vi "LV3Climb.vi"(7 "Deactivate?":bool, 8 "error in (no error)":errorcluster, 9 "Activate?":bool, 10 "Reclimb?":bool, 11 "Elevator Concrete in":refnum<class "Elevator Arm.lvclass">) -> (0 "error out":errorcluster, 1 "activate wrist lock":bool, 3 "Elevator Concrete out":refnum<class "Elevator Arm.lvclass">)   [LabVIEW 2018, in "Elevator.lvlib" / "Elevator Arm.lvclass"]
uses:
  Elevator Arm.lvclass
  C:/Users/Howdy Bots/Documents/2019DeepSpace/Classes/Elevator/Elevator.lvclass
  Controls/Elevator States Climb.ctl
  Elevator.lvclass/Elevator.ctl
  <vilib>/Rock Robotics/WPI/ThirdParty/Phoenix-LabVIEW/Motor Controller/Controls/CTRE_Phoenix_MotorControl_ControlMode.ctl
  Elevator Arm.lvclass/Elevator Arm.ctl
  Public Methods/Read Arm Position Values.vi
  <vilib>/Rock Robotics/WPI/ThirdParty/Phoenix-LabVIEW/Motor Controller/Get/CTRE_Phoenix_MotorController_GetQuadratureData.vi
  <vilib>/Rock Robotics/Network Tables/NT Write String.vi
  Elevator.lvclass
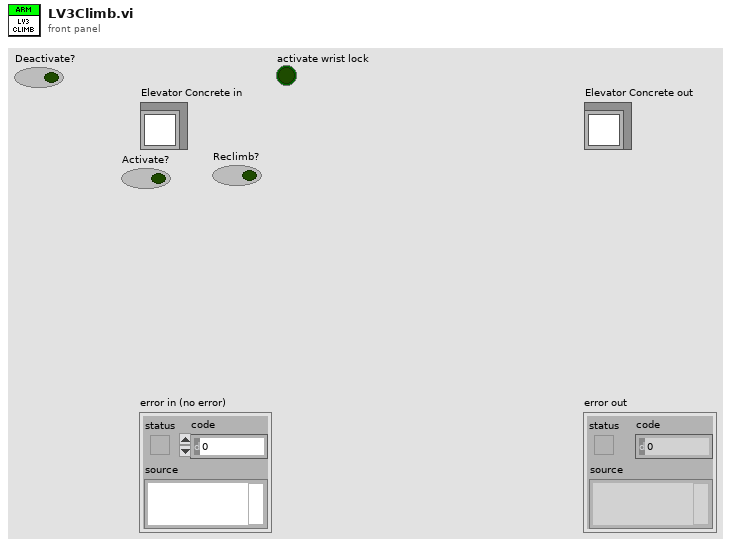
[diagram p1: front panel]
types:
  T1 = typedef "Elevator.lvlib/Elevator.lvclass/Elevator States Climb.ctl" = enum16{"Pre-Lift", "Deploy", "Activate Suction", "Climb", "Climbed", "Unclimb", ""}
  T2 = typedef "Elevator.lvlib/Elevator.lvclass/Elevator Constants.ctl" = cluster{"Arm Motion Magic Max Velocity":u32, "Arm Motion Magic Max Acceleration":u32, "Wrist Motion Magic Max Velocity":u32, "Wrist Motion Magic Max Acceleration":u32, "Elevator Linear Motion Magic Max Velocity":u32, "Elevator Linear Motion Magic Max Acceleration":u32, "Arm Gear Ratio":dbl, "Wrist Gear Ratio":dbl, "Elevator Linear Gear Ratio":dbl, "Arm Encoder ABS Value":i32, "Wrist Encoder ABS Value":i32}
  T3 = typedef "Elevator.lvlib/Elevator.lvclass/Arm Position Values.ctl" = cluster{"C0 Arm":dbl, "C1 Arm":dbl, "C2 Arm":dbl, "H1 Arm":dbl, "H2 Arm":dbl, "C0 Wrist":dbl, "C1 Wrist ":dbl, "C2 Wrist":dbl, "H1 Wrist":dbl, "H2 Wrist":dbl, "Deploy Arm":dbl, "Deploy Wrist":dbl, "Climb Arm":dbl, "Climb Wrist":dbl, "Stowed Arm":dbl, "Stowed Wrist":dbl, "CS":dbl, "C0":dbl, "C1":dbl, "C2":dbl, "C3":dbl, "H0":dbl, "H1":dbl, "H2":dbl}
  T4 = typedef "CTRE_Phoenix_MotorControl_ControlMode.ctl" = u16
  T5 = typedef "WPI_MotorControlDeviceRef.ctl" = cluster{"DeviceStatus":errorcluster, "Type":T6, "PWM":cluster{"PWM Channel":T7, "DeadBand":T8}, "CAN":cluster{"Device Number":u8, "SetOutput VI Ref":variant, "GetOutput VI Ref":variant, "Enable VI Ref":variant, "Disable VI Ref":variant, "Data":variant}, "Invert":bool, "DIO PWM":cluster{"PWM \"Enable\" Channel":T7, "DIOChannel":T9, "PWM Rate":dbl}}
  T6 = typedef "WPI_MotorControlType.ctl" = enum16{"PWM", "CAN", "DIO PWM"}
  T7 = typedef "FPGA_DIOPWMChannel.ctl" = enum8{"PWM 0", "PWM 1", "PWM 2", "PWM 3", "PWM 4", "PWM 5", "PWM 6", "PWM 7", "PWM 8", "PWM 9", "PWM MXP 0", "PWM MXP 1", "PWM MXP 2", "PWM MXP 3", "PWM MXP 4", "PWM MXP 5", "PWM MXP 6", "PWM MXP 7", "PWM MXP 8", "PWM MXP 9", "Invalid"}
  T8 = typedef "WPI_PWMDeadband.ctl" = cluster{"Name":string, "maxPositivePwm":i32, "minPositivePwm":i32, "centerPwm":i32, "maxNegativePwm":i32, "minNegativePwm":i32, "angularRange":u16}
  T9 = typedef "FPGA_DIOChannel.ctl" = enum8{"DIO 0", "DIO 1", "DIO 2", "DIO 3", "DIO 4", "DIO 5", "DIO 6", "DIO 7", "DIO 8", "DIO 9", "DIO MXP 0", "DIO MXP 1", "DIO MXP 2", "DIO MXP 3", "DIO MXP 4", "DIO MXP 5", "DIO MXP 6", "DIO MXP 7", "DIO MXP 8", "DIO MXP 9", "DIO MXP 10", "DIO MXP 11", "DIO MXP 12", "DIO MXP 13", "DIO MXP 14", "DIO MXP 15", "SPI Port CS1", "SPI Port CS2", "SPI Port CS3", "SPI Port MISO", "SPI Port MOSI", "Invalid"}
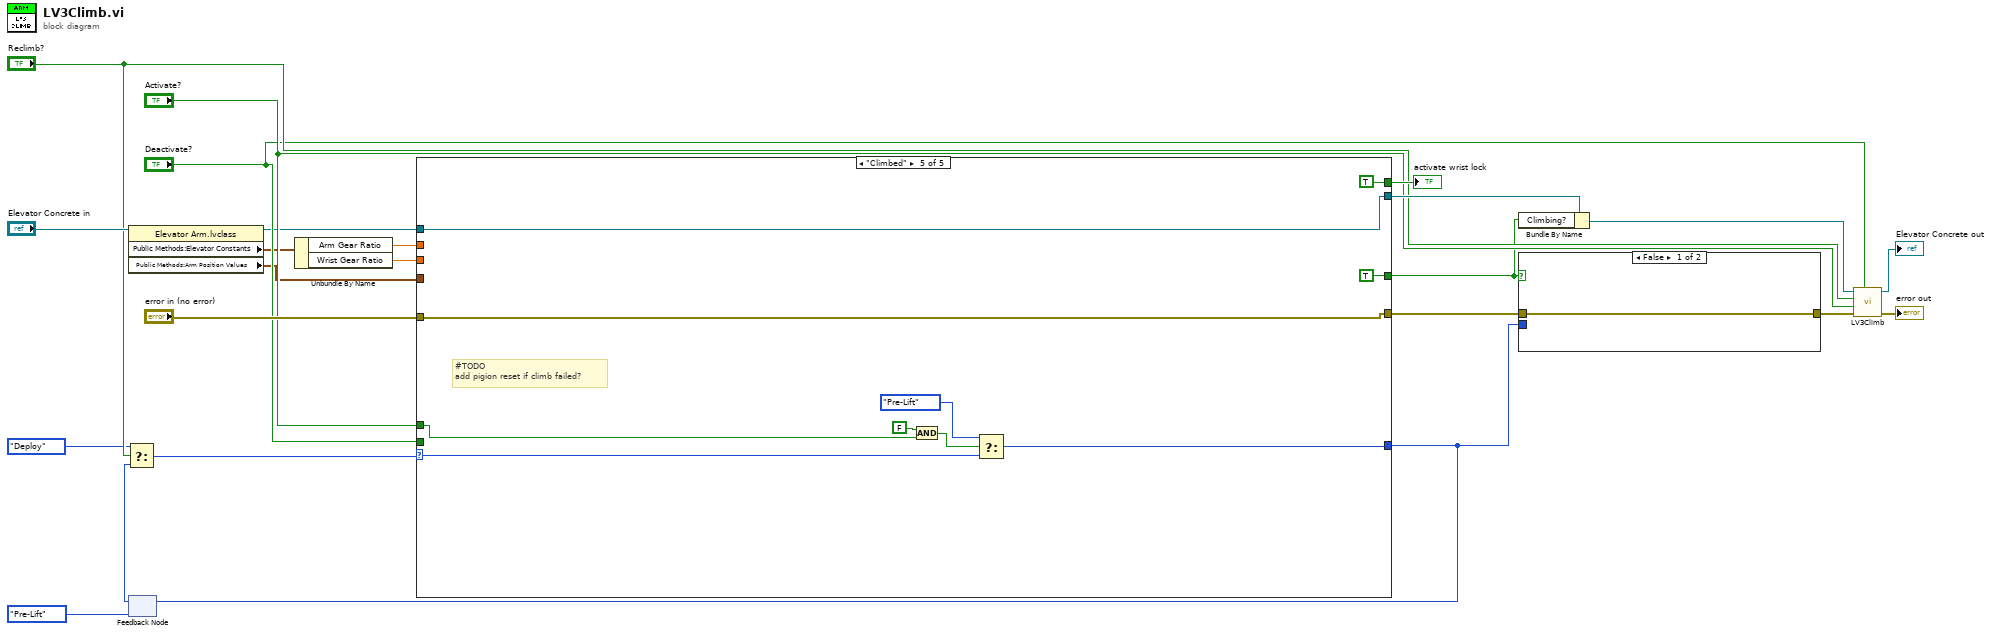
[diagram p0: block diagram]
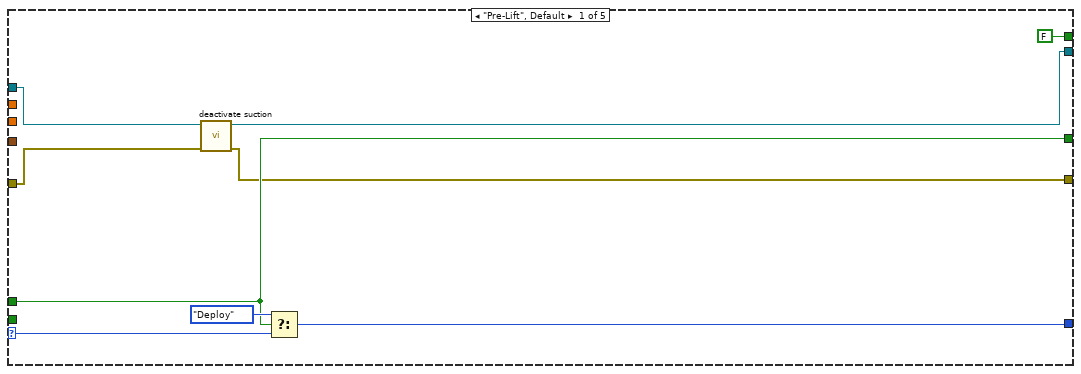
[diagram p2: hidden frame]
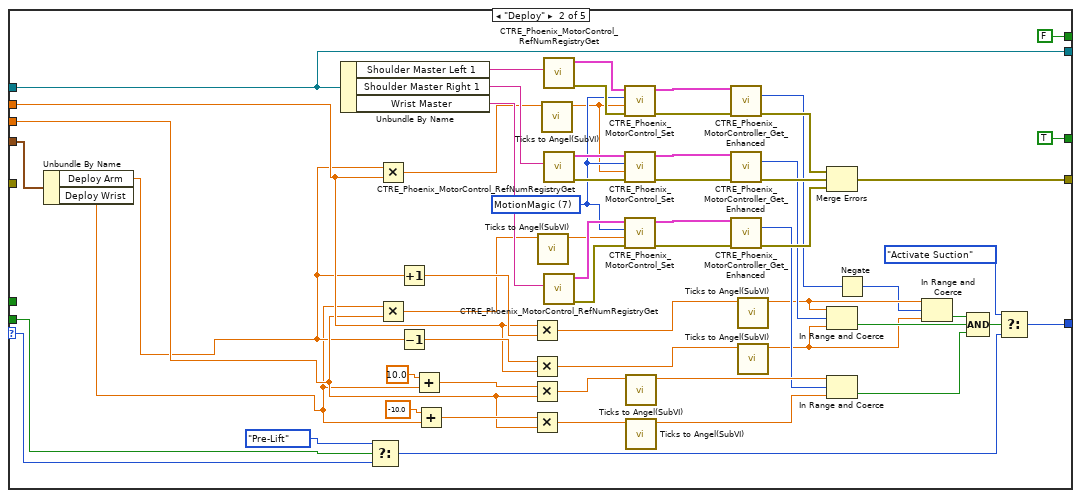
[diagram p3: hidden frame]
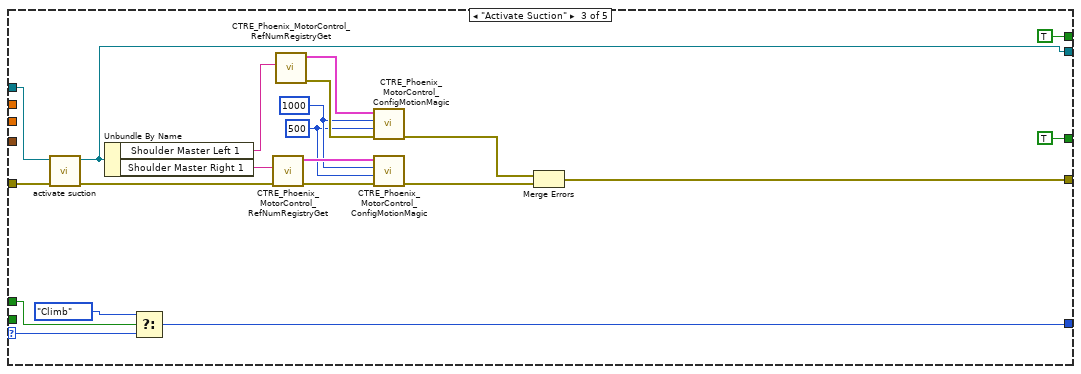
[diagram p4: hidden frame]
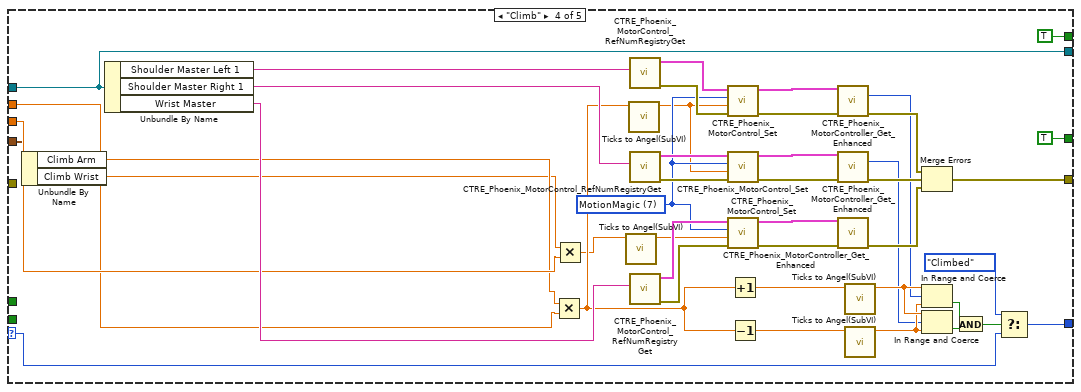
[diagram p5: hidden frame]
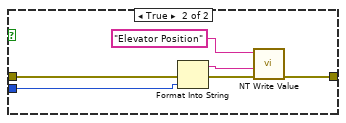
[diagram p6: hidden frame]
diagram:
  n1 = property class="Elevator Arm.lvclass"(reference="Elevator Concrete in") -> (reference out=w5:refnum<class "Elevator Arm.lvclass">, "Public Methods:Elevator Constants"=w3:T2, "Public Methods:Arm Position Values"=w4:T3)  [unwired: 1 in, 1 out]
  n2 = feedback #1(Elevator_States_Climb."Pre-Lift") -> (w13:T1)
  n3 = Select(t=Elevator_States_Climb."Deploy", s="Reclimb?", f=w13) -> (s? t:f=w7:T1)
  n4 = Unbundle By Name(w3) -> ("Arm Gear Ratio"=w2:dbl, "Wrist Gear Ratio"=w1:dbl)
  n5 = case shown="\"Climbed\"" w7 {
    selector: w7 -> [w31 w38 w110 w157 w160]
    tunnel: "Activate?" -> [w29 _ w107 _ w164]
    tunnel: w5 -> [w27 w92 w113 w152 w167]
    tunnel: [w26 w92 w106 w152 w167] -> w22
    tunnel: "error in (no error)" -> [w25 _ w112 _ w166]
    tunnel: [w24 w91 w98 w155 w166] -> w11
    tunnel: [w30 w90 w111 w156 w161] -> w9
    tunnel: [w29 TRUE TRUE TRUE TRUE] -> w8
    tunnel: [FALSE FALSE TRUE TRUE TRUE] -> w19
    tunnel: "Deactivate?" -> [_ w40 _ _ _]
    tunnel: w4 -> [_ w35 _ w116 _]
    tunnel: w2 -> [_ w37 _ w117 _]
    tunnel: w1 -> [_ w36 _ w118 _]
    frame "Pre-Lift", Default {
      n6 = call "deactivate suction.vi"("error in (no error)"=w25, "Elevator Concrete in"=w27) -> ("error out"=w24:errorcluster, "Elevator Concrete out"=w26:refnum<class "Elevator Arm.lvclass">)  [unwired: 8 in]
      n7 = Select(t=Elevator_States_Climb."Deploy", s=w29, f=w31) -> (s? t:f=w30:T1)
    }
    frame "Deploy" {
      w68 = T4 7 items=["PercentOutput"=0, "Position"=1, "Velocity"=2, "Current"=3, "Follower"=5, "MotionProfile"=6, "MotionMagic"=7, "MotionProfileArc"=10, "Disabled"=15] ("Control Mode")
      n8 = Unbundle By Name(w35) -> ("Deploy Arm"=w34:dbl, "Deploy Wrist"=w33:dbl)
      n9 = Unbundle By Name(w92) -> ("Shoulder Master Left 1"=w67:string, "Shoulder Master Right 1"=w82:string, "Wrist Master"=w83:string)
      n10 = Select(t=Elevator_States_Climb."Pre-Lift", s=w40, f=w38) -> (s? t:f=w39:T1)
      n11 = Multiply(x=w34, y=w37) -> (x*y=w45:dbl)
      n12 = Multiply(x=w33, y=w36) -> (x*y=w50:dbl)
      n13 = Increment(x=w34) -> (x+1=w60:dbl)
      n14 = Decrement(x=w34) -> (x-1=w59:dbl)
      n15 = Add(x=10.0, y=w33) -> (x+y=w57:dbl)
      n16 = Add(x=-10.0, y=w33) -> (x+y=w56:dbl)
      n17 = Multiply(x=w37, y=w60) -> (x*y=w43:dbl)
      n18 = Multiply(x=w59, y=w37) -> (x*y=w44:dbl)
      n19 = Multiply(x=w57, y=w36) -> (x*y=w47:dbl)
      n20 = Multiply(x=w56, y=w36) -> (x*y=w46:dbl)
      n21 = call "Ticks to Angel(SubVI).vi"("Numeric in"=w50) -> ("Numeric out"=w73:dbl)  [unwired: 10 in]
      n22 = call "Ticks to Angel(SubVI).vi"("Numeric in"=w45) -> ("Numeric out"=w65:dbl)  [unwired: 10 in]
      n23 = call <vilib>:"CTRE_Phoenix_MotorControl_RefNumRegistryGet.vi"("refnum name"=w67) -> ("error out"=w70:errorcluster, "PhoenixMotorControlDevRef"=w72:T5)  [unwired: 9 in]
      n24 = call <vilib>:"CTRE_Phoenix_MotorControl_RefNumRegistryGet.vi"("refnum name"=w82) -> ("error out"=w87:errorcluster, "PhoenixMotorControlDevRef"=w86:T5)  [unwired: 9 in]
      n25 = call <vilib>:"CTRE_Phoenix_MotorControl_RefNumRegistryGet.vi"("refnum name"=w83) -> ("error out"=w84:errorcluster, "PhoenixMotorControlDevRef"=w85:T5)  [unwired: 9 in]
      n26 = call <vilib>:"CTRE_Phoenix_MotorControl_Set.vi"("error in (no error)"=w70, "Output"=w65, "Control Mode"=w68, "PhoenixMotorControlDevRef"=w72) -> ("error out"=w69:errorcluster, "PhoenixMotorControlDevRef"=w71:T5)  [unwired: 6 in]
      n27 = call <vilib>:"CTRE_Phoenix_MotorControl_Set.vi"("error in (no error)"=w87, "Output"=w65, "Control Mode"=w68, "PhoenixMotorControlDevRef"=w86) -> ("error out"=w77:errorcluster, "PhoenixMotorControlDevRef"=w78:T5)  [unwired: 6 in]
      n28 = call <vilib>:"CTRE_Phoenix_MotorControl_Set.vi"("error in (no error)"=w84, "Output"=w73, "Control Mode"=w68, "PhoenixMotorControlDevRef"=w85) -> ("error out"=w79:errorcluster, "PhoenixMotorControlDevRef"=w80:T5)  [unwired: 6 in]
      n29 = call "Ticks to Angel(SubVI).vi"("Numeric in"=w47) -> ("Numeric out"=w54:dbl)  [unwired: 10 in]
      n30 = call "Ticks to Angel(SubVI).vi"("Numeric in"=w46) -> ("Numeric out"=w55:dbl)  [unwired: 10 in]
      n31 = call-poly <vilib>:"CTRE_Phoenix_MotorController_Get_Enhanced.vi"("PhoenixMotorControlDevRef"=w71, "error in"=w69) -> ("Quadrature Position"=w61:i32, "error out"=w66:errorcluster)  [unwired: 10 in, 2 out]
      n32 = call-poly <vilib>:"CTRE_Phoenix_MotorController_Get_Enhanced.vi"("PhoenixMotorControlDevRef"=w78, "error in"=w77) -> ("Quadrature Position"=w58:i32, "error out"=w75:errorcluster)  [unwired: 10 in, 2 out]
      n33 = call-poly <vilib>:"CTRE_Phoenix_MotorController_Get_Enhanced.vi"("PhoenixMotorControlDevRef"=w80, "error in"=w79) -> ("Quadrature Position"=w53:i32, "error out"=w74:errorcluster)  [unwired: 10 in, 2 out]
      n34 = call "Ticks to Angel(SubVI).vi"("Numeric in"=w43) -> ("Numeric out"=w52:dbl)  [unwired: 10 in]
      n35 = call "Ticks to Angel(SubVI).vi"("Numeric in"=w44) -> ("Numeric out"=w51:dbl)  [unwired: 10 in]
      n36 = Merge Errors(w66, w75, w74) -> (w91:errorcluster)
      n37 = In Range and Coerce(upper limit=w52, x=w58, lower limit=w51) -> (In Range?=w63:bool)  [unwired: 1 out]
      n38 = In Range and Coerce(upper limit=w54, x=w53, lower limit=w55) -> (In Range?=w64:bool)  [unwired: 1 out]
      n39 = Negate(x=w61) -> (-x=w42:i32)
      n40 = In Range and Coerce(upper limit=w52, x=w42, lower limit=w51) -> (In Range?=w62:bool)  [unwired: 1 out]
      n41 = Compound Arithmetic op=AND(w62, w63, w64) -> (w76:bool)
      n42 = Select(t=Elevator_States_Climb."Activate Suction", s=w76, f=w39) -> (s? t:f=w90:T1)
    }
    frame "Activate Suction" {
      w95 = 1000 ("Cruise Velocity")
      w94 = 500 ("Acceleration")
      n43 = call "activate suction.vi"("error in (no error)"=w112, "Elevator Concrete in"=w113) -> ("error out"=w99:errorcluster, "Elevator Concrete out"=w106:refnum<class "Elevator Arm.lvclass">)  [unwired: 8 in]
      n44 = Unbundle By Name(w106) -> ("Shoulder Master Left 1"=w104:string, "Shoulder Master Right 1"=w105:string)
      n45 = Select(t=Elevator_States_Climb."Climb", s=w107, f=w110) -> (s? t:f=w111:T1)
      n46 = call <vilib>:"CTRE_Phoenix_MotorControl_RefNumRegistryGet.vi"("error in (no error)"=w99, "refnum name"=w105) -> ("error out"=w103:errorcluster, "PhoenixMotorControlDevRef"=w102:T5)  [unwired: 8 in]
      n47 = call <vilib>:"CTRE_Phoenix_MotorControl_RefNumRegistryGet.vi"("refnum name"=w104) -> ("error out"=w101:errorcluster, "PhoenixMotorControlDevRef"=w100:T5)  [unwired: 9 in]
      n48 = call <vilib>:"CTRE_Phoenix_MotorControl_ConfigMotionMagic.vi"("error in (no error)"=w101, "Acceleration"=w94, "Cruise Velocity"=w95, "PhoenixMotorControlDevRef"=w100) -> ("error out"=w97:errorcluster)  [unwired: 6 in, 1 out]
      n49 = call <vilib>:"CTRE_Phoenix_MotorControl_ConfigMotionMagic.vi"("error in (no error)"=w103, "Acceleration"=w94, "Cruise Velocity"=w95, "PhoenixMotorControlDevRef"=w102) -> ("error out"=w96:errorcluster)  [unwired: 6 in, 1 out]
      n50 = Merge Errors(w97, w96) -> (w98:errorcluster)
    }
    frame "Climb" {
      w134 = T4 7 items=["PercentOutput"=0, "Position"=1, "Velocity"=2, "Current"=3, "Follower"=5, "MotionProfile"=6, "MotionMagic"=7, "MotionProfileArc"=10, "Disabled"=15] ("Control Mode")
      n51 = Unbundle By Name(w116) -> ("Climb Arm"=w115:dbl, "Climb Wrist"=w114:dbl)
      n52 = Unbundle By Name(w152) -> ("Shoulder Master Left 1"=w133:string, "Shoulder Master Right 1"=w146:string, "Wrist Master"=w147:string)
      n53 = Multiply(x=w115, y=w117) -> (x*y=w120:dbl)
      n54 = Multiply(x=w114, y=w118) -> (x*y=w119:dbl)
      n55 = call "Ticks to Angel(SubVI).vi"("Numeric in"=w119) -> ("Numeric out"=w121:dbl)  [unwired: 10 in]
      n56 = call "Ticks to Angel(SubVI).vi"("Numeric in"=w120) -> ("Numeric out"=w122:dbl)  [unwired: 10 in]
      n57 = call <vilib>:"CTRE_Phoenix_MotorControl_RefNumRegistryGet.vi"("refnum name"=w133) -> ("error out"=w136:errorcluster, "PhoenixMotorControlDevRef"=w138:T5)  [unwired: 9 in]
      n58 = call <vilib>:"CTRE_Phoenix_MotorControl_RefNumRegistryGet.vi"("refnum name"=w146) -> ("error out"=w151:errorcluster, "PhoenixMotorControlDevRef"=w150:T5)  [unwired: 9 in]
      n59 = call <vilib>:"CTRE_Phoenix_MotorControl_RefNumRegistryGet.vi"("refnum name"=w147) -> ("error out"=w148:errorcluster, "PhoenixMotorControlDevRef"=w149:T5)  [unwired: 9 in]
      n60 = call <vilib>:"CTRE_Phoenix_MotorControl_Set.vi"("error in (no error)"=w136, "Output"=w122, "Control Mode"=w134, "PhoenixMotorControlDevRef"=w138) -> ("error out"=w135:errorcluster, "PhoenixMotorControlDevRef"=w137:T5)  [unwired: 6 in]
      n61 = call <vilib>:"CTRE_Phoenix_MotorControl_Set.vi"("error in (no error)"=w151, "Output"=w122, "Control Mode"=w134, "PhoenixMotorControlDevRef"=w150) -> ("error out"=w142:errorcluster, "PhoenixMotorControlDevRef"=w143:T5)  [unwired: 6 in]
      n62 = call <vilib>:"CTRE_Phoenix_MotorControl_Set.vi"("error in (no error)"=w148, "Output"=w121, "Control Mode"=w134, "PhoenixMotorControlDevRef"=w149) -> ("error out"=w144:errorcluster, "PhoenixMotorControlDevRef"=w145:T5)  [unwired: 6 in]
      n63 = Increment(x=w120) -> (x+1=w130:dbl)
      n64 = Decrement(x=w120) -> (x-1=w129:dbl)
      n65 = call-poly <vilib>:"CTRE_Phoenix_MotorController_Get_Enhanced.vi"("PhoenixMotorControlDevRef"=w137, "error in"=w135) -> ("Quadrature Position"=w125:i32, "error out"=w132:errorcluster)  [unwired: 10 in, 2 out]
      n66 = call-poly <vilib>:"CTRE_Phoenix_MotorController_Get_Enhanced.vi"("PhoenixMotorControlDevRef"=w143, "error in"=w142) -> ("Quadrature Position"=w126:i32, "error out"=w140:errorcluster)  [unwired: 10 in, 2 out]
      n67 = call-poly <vilib>:"CTRE_Phoenix_MotorController_Get_Enhanced.vi"("PhoenixMotorControlDevRef"=w145, "error in"=w144) -> ("error out"=w139:errorcluster)  [unwired: 10 in, 3 out]
      n68 = call "Ticks to Angel(SubVI).vi"("Numeric in"=w130) -> ("Numeric out"=w128:dbl)  [unwired: 10 in]
      n69 = call "Ticks to Angel(SubVI).vi"("Numeric in"=w129) -> ("Numeric out"=w127:dbl)  [unwired: 10 in]
      n70 = Merge Errors(w132, w140, w139) -> (w155:errorcluster)
      n71 = In Range and Coerce(upper limit=w128, x=w125, lower limit=w127) -> (In Range?=w123:bool)  [unwired: 1 out]
      n72 = In Range and Coerce(upper limit=w128, x=w126, lower limit=w127) -> (In Range?=w124:bool)  [unwired: 1 out]
      n73 = And(x=w123, y=w124) -> (x .and. y?=w141:bool)
      n74 = Select(t=Elevator_States_Climb."Climbed", s=w141, f=w157) -> (s? t:f=w156:T1)
    }
    frame "Climbed" {
      # "#TODO\nadd pigion reset if climb failed?"
      n75 = And(x=FALSE, y=w164) -> (x .and. y?=w165:bool)
      n76 = Select(t=Elevator_States_Climb."Pre-Lift", s=w165, f=w160) -> (s? t:f=w161:T1)
    }
  }
  "activate wrist lock" <- w19
  n77 = feedback-in #1(w9) -> ()
  n78 = Bundle By Name(cluster=w22, "Climbing?"=w8) -> (w18:refnum<class "Elevator Arm.lvclass">)
  n79 = case shown="False" w8 {
    tunnel: [w168 w171] -> w10
    tunnel: w11 -> [w168 w170]
    tunnel: w9 -> [_ w169]
    frame False {
    }
    frame True {
      n80 = Format Into String(error in=w170, w169) -> (resulting string=w173:string, error out=w172:errorcluster)  [unwired: 2 in]
      n81 = call-poly <vilib>:"NT Write Value.vi"("error in"=w172, "String"=w173, "Name"="Elevator Position") -> ("error out"=w171:errorcluster)  [unwired: 8 in]
    }
  }
  n82 = call-parent "LV3Climb.vi"("Deactivate?"="Deactivate?", "error in (no error)"=w10, "Activate?"="Activate?", "Redeploy?"="Reclimb?", "Elevator in"=w18) -> ("error out"=→"error out":errorcluster, "Elevator out"=→"Elevator Concrete out":refnum<class "Elevator Arm.lvclass">)  [unwired: 4 in, 1 out]
